vi "Get Element.vi"(8 "error in (no error)":errorcluster, 10 "Key":string, 11 "SMO.Dictionary.Variant in":refnum<class "SMO.Dictionary.Variant.lvclass">) -> (0 "error out":errorcluster, 1 "Value":variant, 2 "Key dup":string, 3 "SMO.Dictionary.Variant out":refnum<class "SMO.Dictionary.Variant.lvclass">)   [LabVIEW 2013, in "SMO.Dictionary.lvlib" / "SMO.Dictionary.Variant.lvclass"]
uses:
  SMO.Dictionary.Variant.lvclass
  SMO.Dictionary.Variant.lvclass/SMO.Dictionary.Variant.ctl
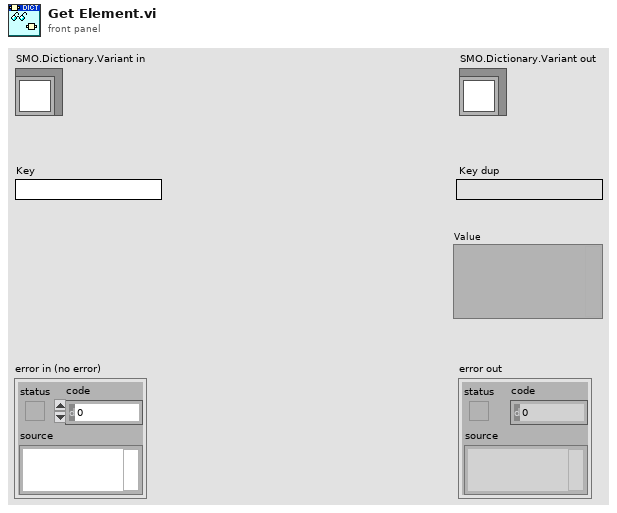
[diagram p1: front panel]
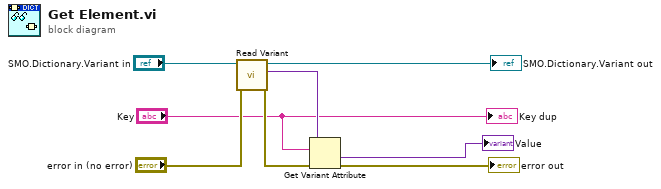
[diagram p0: block diagram]
diagram:
  n1 = call "Read Variant.vi"("error in (no error)"="error in (no error)", "SMO.Dictionary.Variant in"="SMO.Dictionary.Variant in") -> ("error out"=w3:errorcluster, "Variant"=w5:variant, "SMO.Dictionary.Variant out"=→"SMO.Dictionary.Variant out":refnum<class "SMO.Dictionary.Variant.lvclass">)  [unwired: 7 in]
  n2 = Get Variant Attribute(Variant=w5, name="Key", error in=w3) -> (value=→"Value":variant, error out=→"error out":errorcluster)  [unwired: 1 in, 2 out]
  "Key dup" <- "Key"
